vi "get_key_list.vi"(8 "error in (no error)":errorcluster, 11 "Map in":refnum<class "Map.lvclass">) -> (0 "error out":errorcluster, 2 "keys":string[](array[string]), 3 "Map out":refnum<class "Map.lvclass">, 4 "empty?":bool)   [LabVIEW 2010, in "Map.lvclass"]
doc: "This method returns the keys of the key-value pair entries of a map (only for direct child nodes). A boolean indicator shows whether the map is empty or not."
uses:
  Map.lvclass
  Map.lvclass/Map.ctl
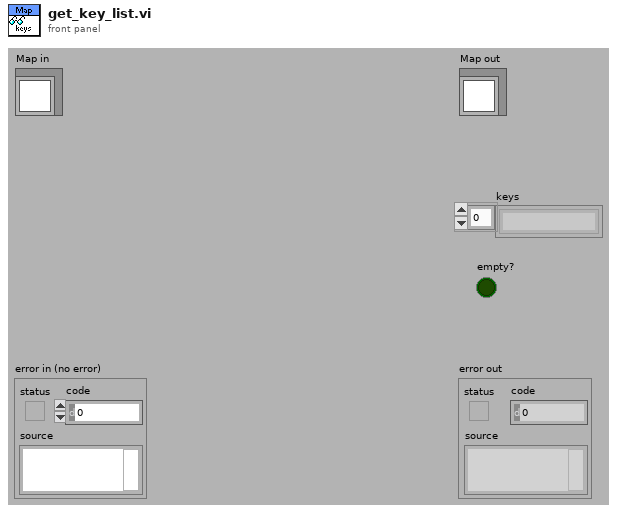
[diagram p1: front panel]
types:
  T1 = typedef "Map.lvclass/element_cluster.ctl" = cluster{"key":string, "value":variant}
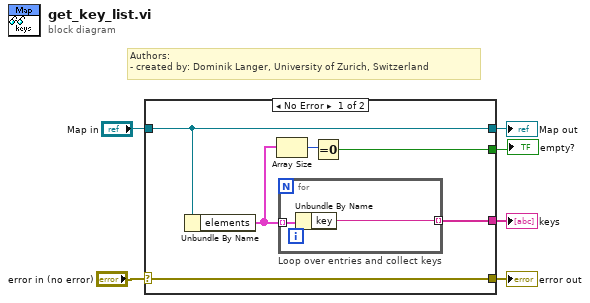
[diagram p0: block diagram]
diagram:
  # "Authors: \n- created by: Dominik Langer, University of Zurich, Switzerland"
  n1 = case shown="No Error" "error in (no error)" {
    selector: "error in (no error)" -> [w12 w16]
    tunnel: [w12 w16] -> w5
    tunnel: [w11 w15] -> w3
    tunnel: "Map in" -> [w11 w15]
    tunnel: [w10 _] -> w2
    tunnel: [w7 _] -> w1
    frame No Error {
      n2 = Unbundle By Name(w11) -> ("elements"=w9:T1[])
      n3 = Array Size(array=w9) -> (size(s)=w8:i32)
      n4 = for "Loop over entries and collect keys" {
        tunnel: w9 -> [w14] mode=indexing
        tunnel: [w13] -> w10 mode=indexing
        n5 = Unbundle By Name(w14) -> ("key"=w13:string)
      }
      n6 = Equal To 0?(x=w8) -> (x = 0?=w7:bool)
    }
    frame Error {
    }
  }
  "error out" <- w5
  "Map out" <- w3
  "keys" <- w2
  "empty?" <- w1
